vi "xijk_template_select_booleans.vi"(11 "Select template":u16) -> (0 "FRET?":bool, 2 "Dual emission?":bool, 4 "Number of fluorophores out":i32, 6 "Light source out":i32)   [LabVIEW 2009]
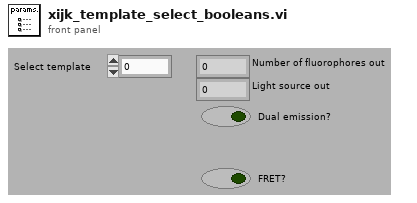
[diagram p1: front panel]
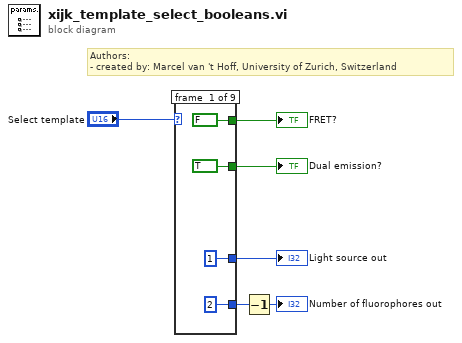
[diagram p0: block diagram]
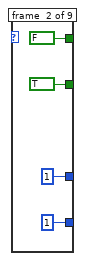
[diagram p2: hidden frame]
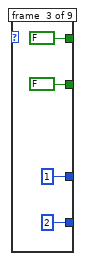
[diagram p3: hidden frame]
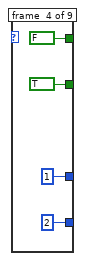
[diagram p4: hidden frame]
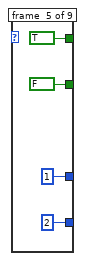
[diagram p5: hidden frame]
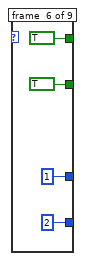
[diagram p6: hidden frame]
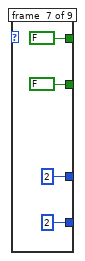
[diagram p7: hidden frame]
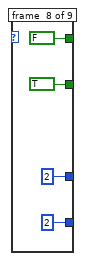
[diagram p8: hidden frame]
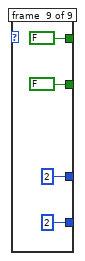
[diagram p9: hidden frame]
diagram:
  # "Authors: \n- created by: Marcel van 't Hoff, University of Zurich, Switzerland"
  n1 = case shown="0, Default" "Select template" {
    tunnel: [FALSE FALSE FALSE FALSE TRUE TRUE FALSE FALSE FALSE] -> w6
    tunnel: [TRUE TRUE FALSE TRUE FALSE TRUE FALSE TRUE FALSE] -> w4
    tunnel: [1 1 1 1 1 1 2 2 2] -> w3
    tunnel: [2 1 2 2 2 2 2 2 2] -> w2
    frame #0 {
    }
    frame #1 {
    }
    frame #2 {
    }
    frame #3 {
    }
    frame #4 {
    }
    frame #5 {
    }
    frame #6 {
    }
    frame #7 {
    }
    frame #8 {
    }
  }
  "FRET?" <- w6
  "Dual emission?" <- w4
  "Light source out" <- w3
  n2 = Decrement(x=w2) -> (x-1=→"Number of fluorophores out":i32)
